vi "Initialize.vi"(7 "Serial Configuration (9600,8,1,N,N)":T1={"Baud Rate"=9600, "Parity"=0, "Data Bits"=8, "Stop Bits"=10, "Flow Control"=0} {"Flow Control" items=["None", "XON/XOFF", "RTS/CTS", "XON/XOFF & RTS/CTS", "DTR/DSR", "XON/XOFF & DTR/DSR"]; "Stop Bits" items=["1.0"=10, "1.5"=15, "2.0"=20]; "Data Bits" items=["7"=7, "8"=8]; "Parity" items=["None", "Odd", "Even", "Mark", "Space"]; "Baud Rate" items=["300"=300, "600"=600, "1200"=1200, "2400"=2400, "4800"=4800, "9600"=9600, "19200"=19200]}, 8 "Error In":errorcluster, 11 "VISA Resource Name":refnum<visa-resource-name>) -> (0 "Error Out":errorcluster, 3 "VISA Resource out":refnum<visa-resource-name>)   [LabVIEW 2014, in "KIT QV.lvlib"]
doc: "This VI opens and configures the VISA interface only.\n\nInstrument ID-Check, Reset and Selftest habe to be performed in the application.\n\nGenerally, you need to call the <b>Initialize</b> VI only once at the beginning of an application."
uses:
  KIT QV.lvlib
panel:
  # "(c) 2015 GSI Helmholtzzentrum für Schwerionenforschung GmbH.  ALL RIGHTS RESERVED."
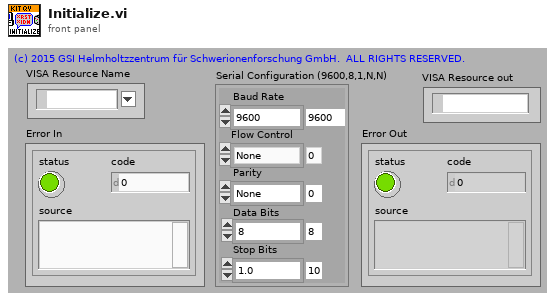
[diagram p1: front panel]
types:
  T1 = cluster{"Baud Rate":u32, "Parity":u16, "Data Bits":u16, "Stop Bits":u16, "Flow Control":u16}
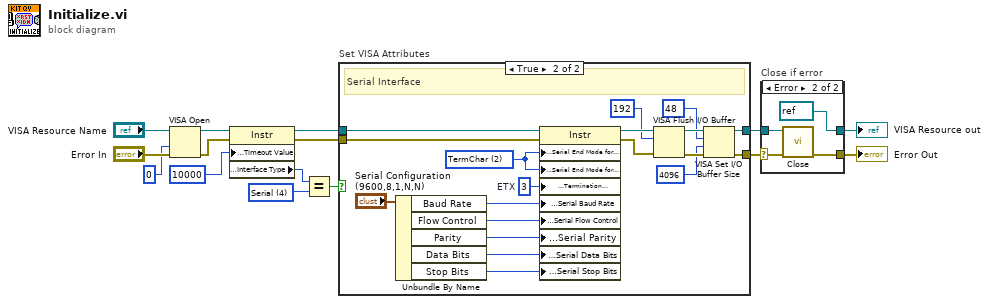
[diagram p0: block diagram]
diagram:
  w8 = u16 4 items=["GPIB"=1, "VXI"=2, "GPIB-VXI"=3, "Serial"=4, "PXI"=5, "TCPIP"=6, "USB"=7] ("Interface Information:Interface Type")
  n1 = VISA Open(access mode=u32 0, error in (no error)="Error In", VISA resource name="VISA Resource Name") -> (VISA resource name=w4:refnum<visa-resource-name>, error out=w3:errorcluster)  [unwired: 2 in]
  n2 = property class="Instr"(reference=w4, error in=w3, "General Settings:Timeout Value"=u32 10000) -> (reference out=w11:refnum<visa-resource-name>, error out=w10:errorcluster, "Interface Information:Interface Type"=w13:u16)
  n3 = Equal?(x=w13, y=w8) -> (x = y?=w9:bool)
  n4 = case "Set VISA Attributes" shown="True" w9 {
    tunnel: [w16 w33] -> w2
    tunnel: [w17 w30] -> w1
    tunnel: w11 -> [w16 w35]
    tunnel: w10 -> [w17 w36]
    frame False {
      # "TCP/IP"
    }
    frame True {
      w18 = u8 3  # ETX
      w25 = u16 2 items=["None", "LastBit", "TermChar"] ("Serial Settings:Serial End Mode for Reads")
      # "Serial Interface"
      n5 = Unbundle By Name("Serial Configuration (9600,8,1,N,N)") -> ("Baud Rate"=w24:u32, "Flow Control"=w20:u16, "Parity"=w22:u16, "Data Bits"=w23:u16, "Stop Bits"=w19:u16)
      n6 = property class="Instr"(reference=w35, error in=w36, "Serial Settings:Serial End Mode for Reads"=w25, "Serial Settings:Serial End Mode for Writes"=w25, "Message Based Settings:Termination Character"=w18, "Serial Settings:Serial Baud Rate"=w24, "Serial Settings:Serial Flow Control"=w20, "Serial Settings:Serial Parity"=w22, "Serial Settings:Serial Data Bits"=w23, "Serial Settings:Serial Stop Bits"=w19) -> (reference out=w29:refnum<visa-resource-name>, error out=w32:errorcluster)
      n7 = VISA Flush I/O Buffer(VISA resource name=w29, mask (16)=u16 192, error in (no error)=w32) -> (VISA resource name out=w34:refnum<visa-resource-name>, error out=w31:errorcluster)
      n8 = VISA Set I/O Buffer Size(VISA resource name=w34, mask (16)=u16 48, size (4096)=u32 4096 ("size (0)"), error in (no error)=w31) -> (VISA resource name out=w33:refnum<visa-resource-name>, error out=w30:errorcluster)
    }
  }
  n9 = case "Close if error" shown="Error" w1 {
    selector: w1 -> [w37 w40]
    tunnel: w2 -> [w38 w41]
    tunnel: [w38 refnum<visa-resource-name> refnum ("VISA resource name out")] -> w6
    tunnel: [w37 w42] -> w5
    frame No Error {
    }
    frame Error {
      n10 = call "Close.vi"("Error In"=w40, "VISA Resource in"=w41) -> ("Error Out"=w42:errorcluster)  [unwired: 9 in]
    }
  }
  "VISA Resource out" <- w6
  "Error Out" <- w5
